vi "LuaVIEW Handle Task Error.vi"(0 "state object ref":T1, 11 "error":errorcluster) -> (4 "cleanup?":bool)   [LabVIEW 2012]
doc: "Handle task execution errors. This removes some non-contended diagram code from the task state machine, thereby saving a bit of memory for each task instance."
uses:
  typedefs/t_LuaVIEW Task State Pane.ctl
  typedefs/t_LuaVIEW Task State Methods.ctl
  typedefs/t_LuaVIEW Task Signals.ctl
  typedefs/t_LuaVIEW Task List Methods.ctl
  library/glb_Library Configuration Globals.vi
  glb_LuaVIEW Configuration Globals.vi
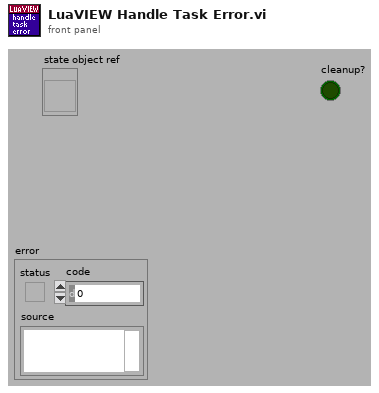
[diagram p1: front panel]
types:
  T1 = typedef "t_LuaVIEW Task State Pane.ctl" = refnum<vi>
  T2 = typedef "t_LuaVIEW Task State Methods.ctl" = enum16{"cleanup", "set initial", "set mode", "set active mode", "set error", "get task info", "get script info", "set signal", "clear signal", "test handled", "test delegated", "test signal", "handle signal", "delegate signal", "allow signal", "disallow signal", "disallow all", "signals?", "delegated signals?", "protection++", "protection--", "protection=0", "message", "next message", "pop message", "message available?", "force stop", "set swap preps", "apply swap preps"}
  T3 = typedef "t_LuaVIEW Task Signals.ctl" = enum32{"resume", "pause", "swap", "stop", "confirm"}
  T4 = typedef "LuaVIEW Task Info.ctl" = cluster{"main script":string, "identifier":string, "class":string, "description":string, "mode":T5, "handler":string, "LuaVIEW reference":T6, "scripts":i32, "hide":bool, "active":bool, "error msg":string, "defer":bool, "launch":enum16{"asynchronous", "manual", "synchronous"}, "main path valid":bool, "start time":dbl, "swap time":dbl, "task VI":refnum<vi>, "prefsys":enum32{"invalid execution system", "user interface", "standard", "instrument i/o", "data acquisition", "other 1", "other 2", "same as caller"}, "priority":enum32{"invalid priority", "background priority", "normal priority", "above normal priority", "high priority", "time critical priority", "subroutine"}, "signal flags":u32, "allow mask":u32, "handle mask":u32, "disallow manual":bool}
  T5 = typedef "t_LuaVIEW Task Modes.ctl" = enum16{"initializing", "running", "executing", "paused", "error", "swapping"}
  T6 = typedef "t_LuaVIEW Reference.ctl" = refnum<k1>
  T7 = typedef "t_LuaVIEW Task List Methods.ctl" = enum16{"clear list", "add", "test", "remove", "get ref", "get task info", "get list", "get script info", "ongoing?", "resume", "pause", "stop", "confirm", "message"}
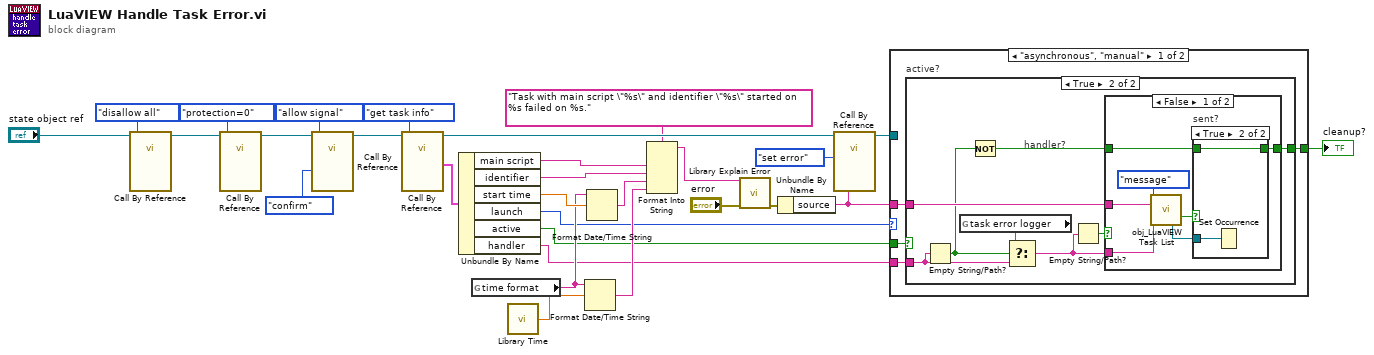
[diagram p0: block diagram]
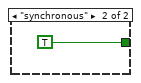
[diagram p5: hidden frame]
diagram:
  n1 = call-by-ref "?"(reference="state object ref", "method"=t_LuaVIEW_Task_State_Methods."disallow all") -> (reference out=w22:T1)  [unwired: 11 in, 6 out]
  n2 = call-by-ref "?"(reference=w22, "method"=t_LuaVIEW_Task_State_Methods."protection=0") -> (reference out=w26:T1)  [unwired: 11 in, 6 out]
  n3 = call-by-ref "?"(reference=w26, "method"=t_LuaVIEW_Task_State_Methods."allow signal", "signal"=t_LuaVIEW_Task_Signals."confirm") -> (reference out=w19:T1)  [unwired: 10 in, 6 out]
  n4 = call-by-ref "?"(reference=w19, "method"=t_LuaVIEW_Task_State_Methods."get task info") -> (reference out=w27:T1, "task info {get task info}"=w28:T4)  [unwired: 11 in, 5 out]
  n5 = Unbundle By Name(w28) -> ("main script"=w13:string, "identifier"=w12:string, "start time"=w17:dbl, "launch"=w5:enum16{"asynchronous", "manual", "synchronous"}, "active"=w1:bool, "handler"=w2:string)
  n6 = global read "glb_Library Configuration Globals.vi" "time format"() -> (w16:string)
  n7 = call "Library Time.vi"() -> ("time"=w18:dbl)  [unwired: 1 in]
  n8 = Format Date/Time String(time format string (%c)=w16, seconds (now)=w18) -> (date/time string=w10:string)  [unwired: 1 in]
  n9 = Format Date/Time String(time format string (%c)=w16, seconds (now)=w17) -> (date/time string=w11:string)  [unwired: 1 in]
  n10 = Format Into String(format string="Task with main script \"%s\" and identifier \"%s\" started on %s failed on %s.", w13, w12, w11, w10) -> (resulting string=w9:string)  [unwired: 2 in, 1 out]
  n11 = call "Library Explain Error.vi"("explanation prefix (none)"=w9, "error in (no error)"="error") -> ("explained error"=w7:errorcluster)  [unwired: 13 in]
  n12 = Unbundle By Name(w7) -> ("source"=w6:string)
  n13 = call-by-ref "?"(reference=w27, "method"=t_LuaVIEW_Task_State_Methods."set error", "string in"=w6) -> (reference out=w4:T1)  [unwired: 10 in, 6 out]
  n14 = case shown="\"asynchronous\", \"manual\"" w5 {
    tunnel: w6 -> [w33 _]
    tunnel: w4 -> [_ _]
    tunnel: [w31 TRUE] -> w3
    tunnel: w2 -> [w32 _]
    tunnel: w1 -> [w30 _]
    frame "asynchronous", "manual" {
      n15 = case "active?" shown="True" w30 {
        tunnel: w33 -> [_ w41]
        tunnel: w32 -> [_ w39]
        tunnel: [_ w35] -> w31
        frame False {
          # "Allow \"Run Task\" to detect\nand return the error when\nit occurred while not\nactive yet (still initializing)."
        }
        frame True {
          # "handler?"
          n16 = Empty String/Path?(string/path=w39) -> (empty?=w36:bool)
          n17 = global read "glb_LuaVIEW Configuration Globals.vi" "task error logger"() -> (w38:string)
          n18 = Not(x=w36) -> (.not. x?=w34:bool)
          n19 = Select(t=w38, s=w36, f=w39) -> (s? t:f=w37:string)
          n20 = Empty String/Path?(string/path=w37) -> (empty?=w40:bool)
          n21 = case shown="False" w40 {
            tunnel: w37 -> [w45 _]
            tunnel: w41 -> [w44 _]
            tunnel: [w43 _] -> w35
            tunnel: w34 -> [w42 _]
            frame False {
              n22 = call "obj_LuaVIEW Task List.vi"("method"=t_LuaVIEW_Task_List_Methods."message", "message"=w44, "task identifier"=w45) -> ("set/ongoing"=w47:bool, "wakeup occurrence"=w48:refnum<k4>)  [unwired: 7 in, 4 out]
              n23 = case "sent?" shown="True" w47 {
                tunnel: w48 -> [_ w50]
                tunnel: w42 -> [_ w49]
                tunnel: [_ w49] -> w43
                frame False {
                }
                frame True {
                  n24 = Set Occurrence(w50) -> ()
                }
              }
            }
            frame True {
            }
          }
        }
      }
    }
    frame "synchronous" {
    }
  }
  "cleanup?" <- w3
